vi "ChazMoveMono.vi"(7 "Monochromator":T1={"Type"=enum."Oriel", "Wavelength (nm)"=500.0, "Wavelength (nm)"="500nm", "Grating, gr/mm"=2, "Grating mode"=enum."IR", "Spectrum mode"={"Spectrum mode?"=FALSE, "Start wavelength (nm)"=0.0, "End wavelength (nm)"=0.0, "Wavelength step (nm)"=0.0, "Wavelength array"=[], "array index"=0}, "VISA"={"delay before read (ms)"=1000, "Mono 1"={"Enable Termination Char (T)"=FALSE, "timeout (msec)"=1000, "Resource name"="COM1", "baud rate"=9600, "data bits"=8, "parity"=0, "stop bits"=10, "flow control"=0}, "Mono 2"={"Enable Termination Char (T)"=FALSE, "timeout (msec)"=1000, "Resource name"="COM1", "baud rate"=9600, "data bits"=8, "parity"=0, "stop bits"=10, "flow control"=0}}} {"VISA"."Mono 2"."flow control" items=["None"=0, "XON/XOFF"=1, "RTS/CTS"=2, "DTR/DSR"=4]; "VISA"."Mono 2"."stop bits" items=["None"=0, "XON/XOFF"=1, "RTS/CTS"=2, "DTR/DSR"=4]; "VISA"."Mono 2"."parity" items=["1.0"=10, "1.5"=15, "2.0"=20]; "VISA"."Mono 1"."flow control" items=["None"=0, "XON/XOFF"=1, "RTS/CTS"=2, "DTR/DSR"=4]; "VISA"."Mono 1"."stop bits" items=["None"=0, "XON/XOFF"=1, "RTS/CTS"=2, "DTR/DSR"=4]; "VISA"."Mono 1"."parity" items=["1.0"=10, "1.5"=15, "2.0"=20]; "Grating, gr/mm" items=["2400", "1800", "1200", "600", "300", "150"]}, 8 "Move to":dbl=2.0, 11 "Current":dbl=2.0) -> (0 "error?":bool, 3 "error? 2":bool)   [LabVIEW 2017]
uses:
  Controls/Params.ctl
  Monochromator.lvlib
  Controls/VISA parameters.ctl
  Serial comms/Serial comms.lvlib
  Controls/Grating.ctl
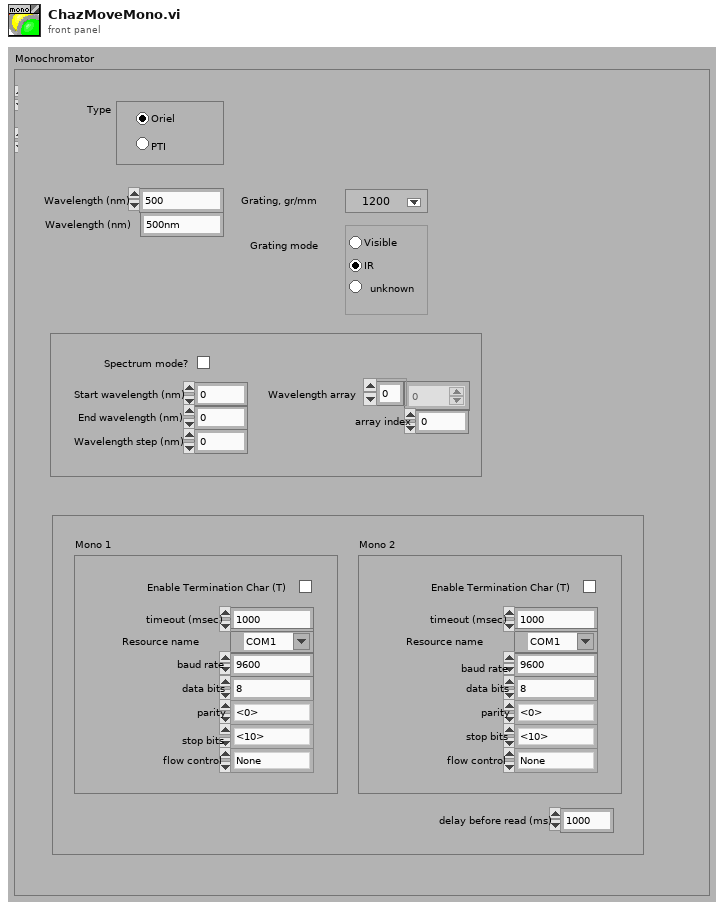
[diagram p1: front panel]
types:
  T1 = typedef "Monochromator.lvlib/Params.ctl" = cluster{"Type":enum32{"Oriel", "PTI"}, "Wavelength (nm)":dbl, "Wavelength (nm)":string, "Grating, gr/mm":u16, "Grating mode":T2, "Spectrum mode":cluster{"Spectrum mode?":bool, "Start wavelength (nm)":dbl, "End wavelength (nm)":dbl, "Wavelength step (nm)":dbl, "Wavelength array":dbl[], "array index":u32}, "VISA":cluster{"delay before read (ms)":u32, "Mono 1":T3, "Mono 2":T3}}
  T2 = typedef "Monochromator.lvlib/Grating.ctl" = enum32{"unknown", "Visible", "IR"}
  T3 = typedef "Serial comms.lvlib/VISA parameters.ctl" = cluster{"Enable Termination Char (T)":bool, "timeout (msec)":u32, "Resource name":refnum<visa-resource-name>, "baud rate":u32, "data bits":u16, "parity":u16, "stop bits":u16, "flow control":u16}
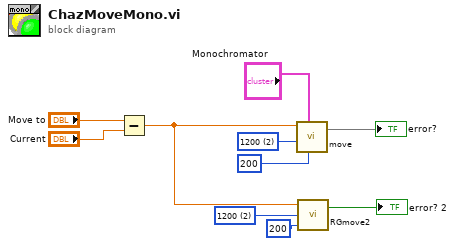
[diagram p0: block diagram]
diagram:
  w6 = u16 2 items=["2400", "1800", "1200", "600", "300", "150"] ("Grating, gr/mm")
  w7 = u16 2 items=["2400", "1800", "1200", "600", "300", "150"] ("Grating, gr/mm")
  n1 = Subtract(x="Move to", y="Current") -> (x-y=w10:dbl)
  n2 = call "move.vi"("delay before read (ms)"=200, 7:"Monochromator", "Grating, gr/mm"=w6, "Wavelength, nm"=w10) -> (5:→"error?")  [unwired: 6 in, 1 out]
  n3 = call "RGmove2.vi"("delay before read (ms)"=200, "Grating, gr/mm"=w7, "Wavelength, nm"=w10) -> ("error?"=→"error? 2":bool)  [unwired: 1 in]
